vi "Test.vi"() -> ()   [LabVIEW 2018]
doc: "This VI is called when test mode begins, and will automatically be terminated when it ends. You can add manual or automatic tests and invoke them from the dashboard."
uses:
  Classes/Joysticks/Joysticks.lvclass/Joysticks.ctl
  Classes/Joysticks/Public Methods/Write Sensitivity(x).vi
  Classes/Joysticks/Public Methods/Write Sensitivity(y).vi
  RobotGlobal.vi
  Classes/Drive/Drive.lvclass
  Classes/Joysticks/Joysticks.lvclass
  Classes/Elevator/Elevator.lvclass
panel:
  in  "Sensitivity(y)":dbl(slide) scale=0.0..1.0
  in  "sensitivity (x)":dbl(slide) scale=0.0..1.0
  in  "finish 2":bool
  in  "update values":bool
  in  "shoulder":dbl
  in  "wrist":dbl
  in  "finish":bool
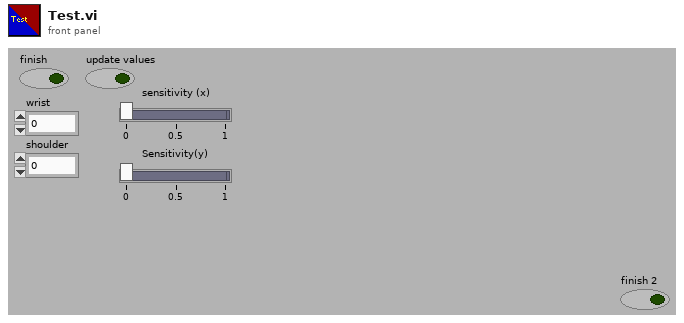
[diagram p1: front panel]
types:
  T1 = typedef "RobotObjects.ctl" = cluster{"Drive.lvclass":refnum<class "Drive.lvclass">, "Pneumatics.lvclass":refnum<class "Pneumatics.lvclass">, "Vision.lvclass":refnum<class "Vision.lvclass">, "Joysticks.lvclass":refnum<class "Joysticks.lvclass">, "Elevator.lvclass":refnum<class "Elevator.lvclass">, "Hatch.lvclass":refnum<class "Hatch.lvclass">, "Cargo.lvclass":refnum<class "Cargo.lvclass">}
  T2 = typedef "Joysticks.lvlib/Joysticks.lvclass/JoystickData.ctl" = cluster{"X Axis":dbl, "Y Axis":dbl, "Drivetrain Shifter (Hold)":bool, "Beak (Toggle)":bool, "Cargo In (Hold)":bool, "Cargo Out (Hold)":bool, "Switch to hatch(toggle)":bool, "Switch to cargo(toggle)":bool, "Elevator Up (Toggle)":bool, "Elevator Down (Toggle)":bool, "AutoDeliver (Hold)":bool, "Climb(toggle)":bool, "Disengage Climb(toggle)":bool}
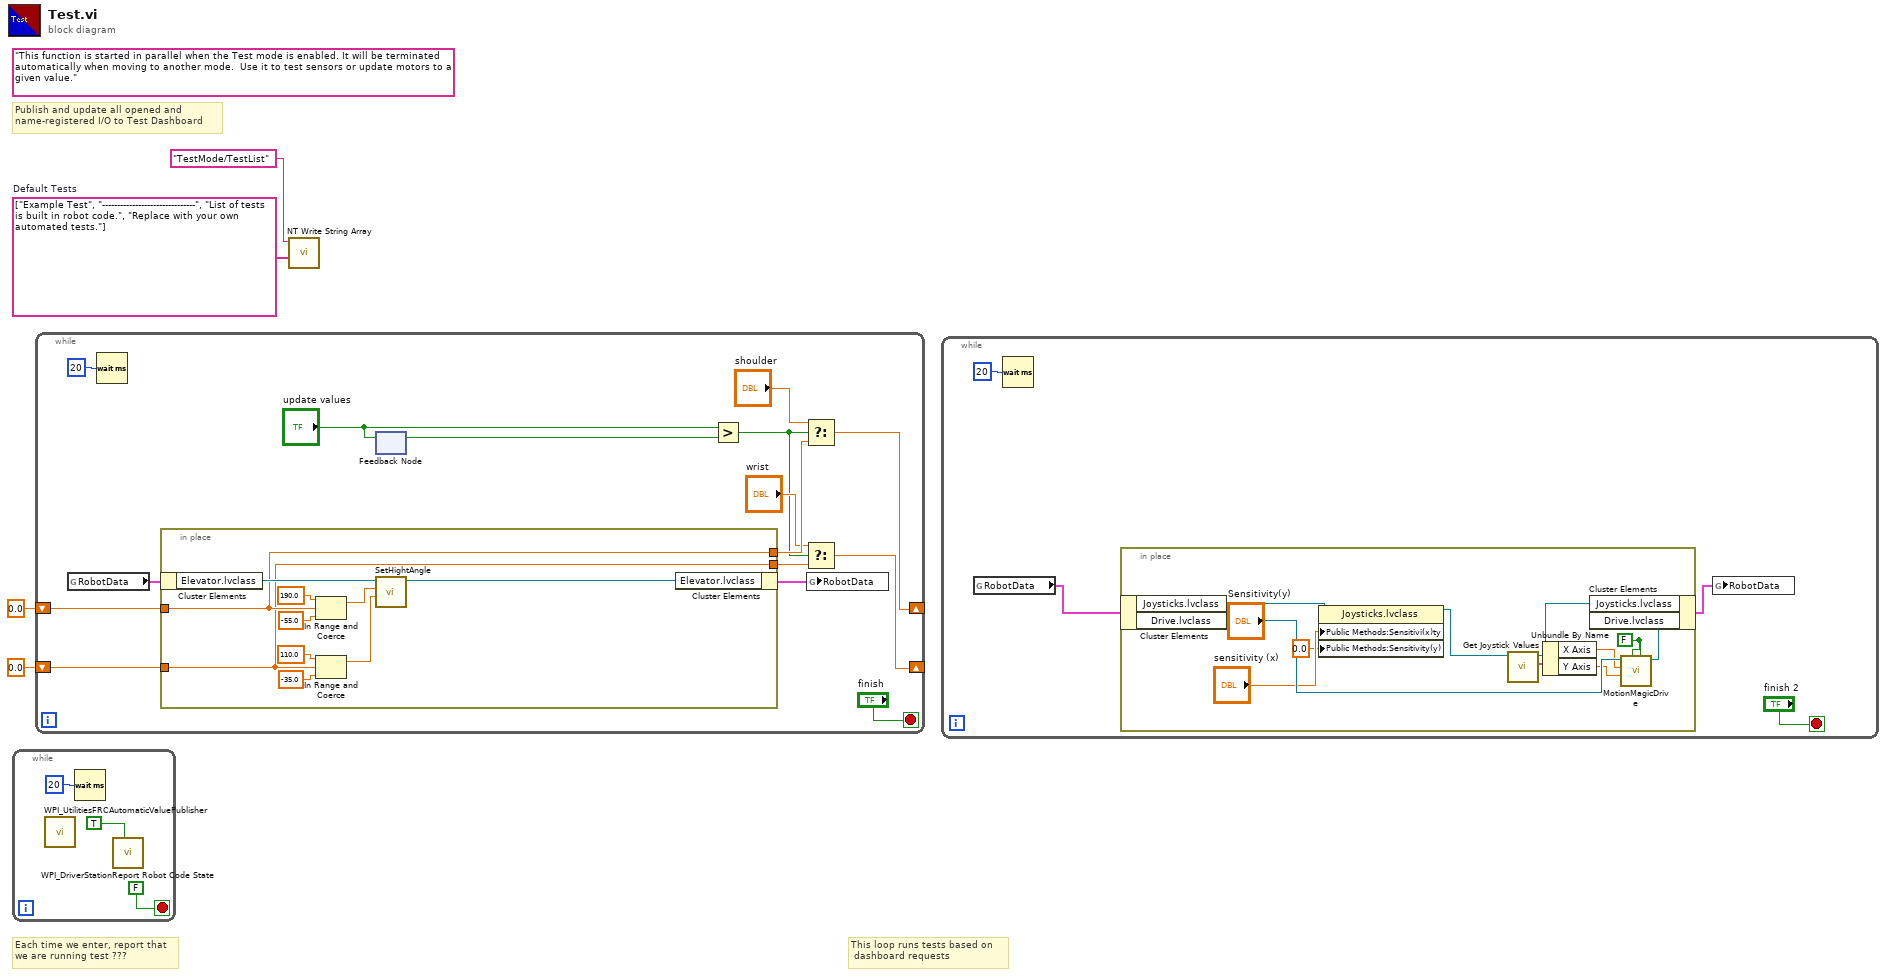
[diagram p0: block diagram]
diagram:
  w4 = string[] ["Example Test", "-------------------------------", "List of tests is built in robot code.", "Replace with your own automated tests."]  # Default Tests
  (unwired) "This function is started in parallel when the Test mode is enabled. It will be terminated automatically when moving to another mode.  Use it to test sensors or update motors to a given value."
  # "This loop runs tests based on \n dashboard requests"
  # "Publish and update all opened and\nname-registered I/O to Test Dashboard"
  # "Each time we enter, report that\nwe are running test ???"
  n1 = while {
    stop <- FALSE stop-if-true
    n2 = call <vilib>:"WPI_UtilitiesFRCAutomaticValuePublisher.vi"() -> ()  [unwired: 12 in]
    n3 = Wait (ms)(milliseconds to wait=u32 20) -> ()  [unwired: 1 out]
    n4 = call <vilib>:"WPI_DriverStationReport Robot Code State.vi"("Test"=TRUE ("Autonomous")) -> ()  [unwired: 10 in, 1 out]
  }
  n5 = while {
    shift-right: [w13] -> _
    shift-left: 0.0 -> [w17]
    shift-right: [w15] -> _
    shift-left: 0.0 -> [w18]
    stop <- "finish" stop-if-true
    n6 = global read "RobotGlobal.vi" "RobotData"() -> (w20:T1)
    n7 = Wait (ms)(milliseconds to wait=u32 20) -> ()  [unwired: 1 out]
    n8 = in-place {
      in-place-border: w18 -> [w30]
      in-place-border: w17 -> [w27]
      in-place-border: [w27] -> w14
      in-place-border: [w30] -> w16
      n9 = in-place-cluster #1(w20) -> ("Elevator.lvclass"=w32:refnum<class "Elevator.lvclass">)
      n10 = In Range and Coerce(upper limit=190.0, x=w30, lower limit=-55.0) -> (coerced(x)=w29:dbl)  [unwired: 1 out]
      n11 = In Range and Coerce(upper limit=110.0, x=w27, lower limit=-35.0) -> (coerced(x)=w28:dbl)  [unwired: 1 out]
      n12 = call-dynamic "SetHightAngle.vi"("Wrist (degrees)"=w28, "Main arm(degrees)"=w29, "Elevator in"=w32) -> ("Elevator out"=w31:refnum<class "Elevator.lvclass">)  [unwired: 7 in, 1 out]
      n13 = in-place-cluster #1("Elevator.lvclass"=w31) -> (w19:T1)
    }
    n14 = feedback #2() -> (w10:bool)  [unwired: 1 in]
    n15 = feedback-in #2("update values") -> ()
    n16 = Greater?(x="update values", y=w10) -> (0:w8:bool)
    n17 = Select(t="shoulder", s=w8, f=w16) -> (s? t:f=w15:dbl)
    n18 = Select(t="wrist", s=w8, f=w14) -> (s? t:f=w13:dbl)
    n19 = global write "RobotGlobal.vi" "RobotData"(w19) -> ()
  }
  n20 = call <vilib>:"NT Write String Array.vi"("String Array"=w4, "Name"="TestMode/TestList") -> ()  [unwired: 9 in, 1 out]
  n21 = while {
    stop <- "finish 2" stop-if-true
    n22 = global read "RobotGlobal.vi" "RobotData"() -> (w34:T1)
    n23 = Wait (ms)(milliseconds to wait=u32 20) -> ()  [unwired: 1 out]
    n24 = in-place {
      w41 = FALSE
      n25 = in-place-cluster #3(w34) -> ("Joysticks.lvclass"=w47:refnum<class "Joysticks.lvclass">, "Drive.lvclass"=w44:refnum<class "Drive.lvclass">)
      n26 = property class="Joysticks.lvclass"(reference=w47, "Public Methods:Sensitivi(x)ty"="sensitivity (x)", "Public Methods:Sensitivity(y)"=0.0 ("Sensitivity(y)")) -> (reference out=w46:refnum<class "Joysticks.lvclass">)  [unwired: 1 in, 1 out]
      n27 = call-dynamic "Get Joystick Values.vi"("Joysticks in"=w46) -> ("Joystick Data"=w45:T2, "Joysticks out"=w39:refnum<class "Joysticks.lvclass">)  [unwired: 8 in, 1 out]
      n28 = Unbundle By Name(w45) -> ("X Axis"=w43:dbl, "Y Axis"=w42:dbl)
      n29 = call-dynamic "MotionMagicDrive.vi"("High gear?"=w41, "Enable Vision"=w41, "Y Axis"=w42, "X Axis"=w43, "Drive in"=w44) -> ("Drive out"=w40:refnum<class "Drive.lvclass">)  [unwired: 5 in, 1 out]
      n30 = in-place-cluster #3("Joysticks.lvclass"=w39, "Drive.lvclass"=w40) -> (w33:T1)
    }
    n31 = global write "RobotGlobal.vi" "RobotData"(w33) -> ()
  }
